vi "Measure.vi"(6 "error in (no error)":errorcluster, 8 "Array of Measurement to Write":dbl[](array[numeric]), 9 "Fluke 2625A (Hydra II) in":refnum<class "Fluke 2625A (Hydra II).lvclass">) -> (0 "error out":errorcluster, 2 "Array of Measurement":dbl[](array[numeric]), 3 "Fluke 2625A (Hydra II) out":refnum<class "Fluke 2625A (Hydra II).lvclass">)   [LabVIEW 2013, in "Generic Data Logger.lvlib" / "Fluke 2625A (Hydra II).lvlib" / "Fluke 2625A (Hydra II).lvclass"]
uses:
  Fluke 2625A (Hydra II).lvclass
  Generic Data Logger Class/Generic Data Logger.lvclass
  <instrlib>/Fluke 2625A/Fluke 2625A.lvlib
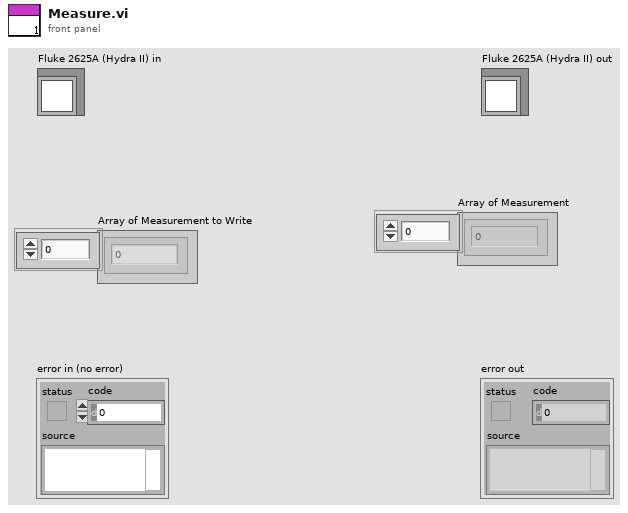
[diagram p1: front panel]
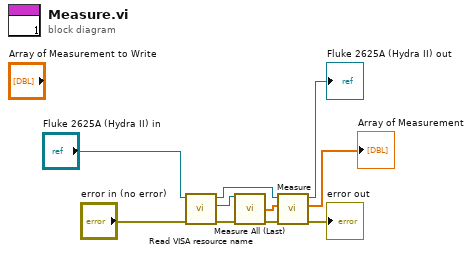
[diagram p0: block diagram]
diagram:
  n1 = call-dynamic "Read VISA resource name.vi"("error in (no error)"="error in (no error)", "Generic Instrument in"="Fluke 2625A (Hydra II) in") -> ("error out"=w4:errorcluster, "VISA resource name"=w5:refnum<visa-resource-name>, "Generic Instrument out"=w6:refnum<class "Fluke 2625A (Hydra II).lvclass">)  [unwired: 7 in]
  n2 = call <instrlib>:"Measure All (Last).vi"("VISA resource name out"=w5, "error in (no error)"=w4) -> ("Numeric Array"=w1:dbl[], "error out 2"=w2:errorcluster)  [unwired: 9 in, 3 out]
  n3 = call-parent "Measure.vi"("error in (no error)"=w2, "Array of Measurement to Write"=w1, "Generic Data Logger in"=w6) -> ("error out"=→"error out":errorcluster, "Array of Measurement"=→"Array of Measurement":dbl[], "Generic Data Logger out"=→"Fluke 2625A (Hydra II) out":refnum<class "Fluke 2625A (Hydra II).lvclass">)  [unwired: 4 in]
